vi "test data setting.vi"() -> ()   [LabVIEW 2017]
uses:
  Controls/dsf channel.ctl
  DSFConfiguration.lvclass
  DSFConfiguration.lvclass/DSFConfiguration.ctl
  DSFChannel/DSFChannel.lvclass/DSFChannel.ctl
  DSFChannel/Read channel info.vi
  Read channels.vi
  DSFChannel/DSFChannel.lvclass
panel:
  out "JSON string":string
  out "Array":T1[](array[typedef])
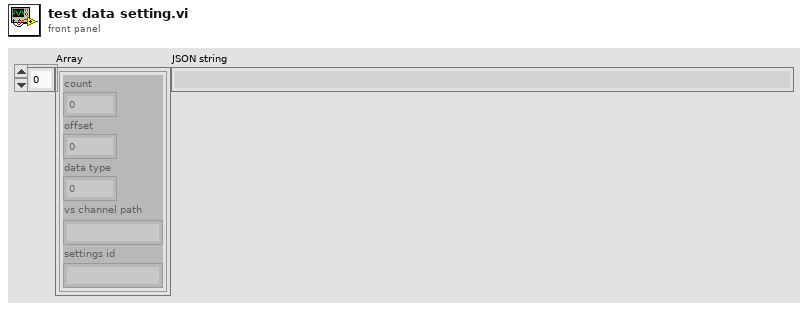
[diagram p1: front panel]
types:
  T1 = typedef "dsf channel.ctl" = cluster{"count":i32, "offset":i32, "data type":i32, "vs channel path":string, "settings id":string}
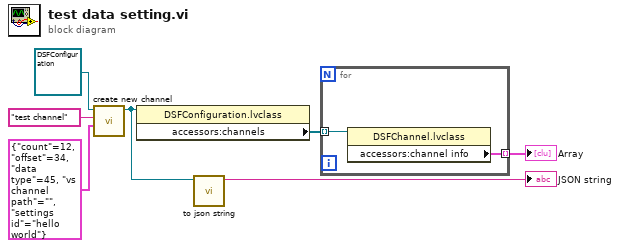
[diagram p0: block diagram]
diagram:
  n1 = call "create new channel.vi"("channel info"=T1 {"count"=12, "offset"=34, "data type"=45, "vs channel path"="", "settings id"="hello world"}, "id"="test channel", "DSFConfiguration in"=refnum<class "DSFConfiguration.lvclass"> refnum ("DSFConfiguration.lvclass")) -> ("DSFConfiguration out"=w3:refnum<class "DSFConfiguration.lvclass">)  [unwired: 7 in, 1 out]
  n2 = property class="DSFConfiguration.lvclass"(reference=w3) -> ("accessors:channels"=w5:refnum<class "DSFChannel.lvclass">[])  [unwired: 1 in, 2 out]
  n3 = call "to json string.vi"("DSFConfiguration.lvclass"=w3) -> ("JSON string"=→"JSON string":string)  [unwired: 10 in]
  n4 = for {
    tunnel: w5 -> [w9] mode=indexing
    tunnel: [w8] -> w4 mode=indexing
    n5 = property class="DSFChannel.lvclass"(reference=w9) -> ("accessors:channel info"=w8:T1)  [unwired: 1 in, 2 out]
  }
  "Array" <- w4
